vi "Get.vi"(9 "Idx (0)":i32, 10 "key":string, 11 "Keys":map{string, string[]}(c390)) -> (0 "Values out":string[](array[string]), 1 "Value out":string, 2 "Found?":bool)   [LabVIEW 2021, in "HttpServer.lvlib"]
uses:
  HttpServer.lvlib
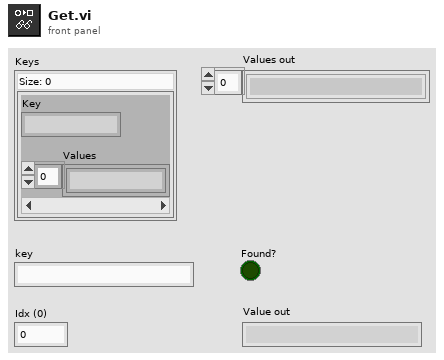
[diagram p1: front panel]
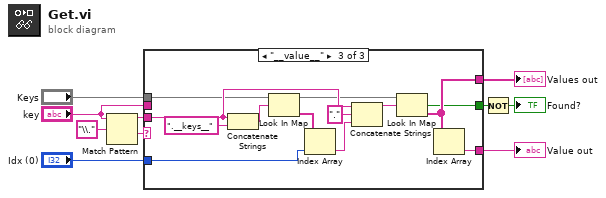
[diagram p0: block diagram]
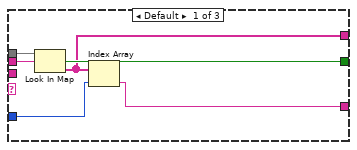
[diagram p2: hidden frame]
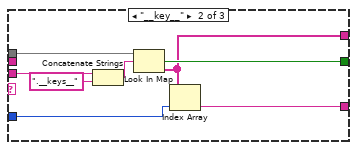
[diagram p3: hidden frame]
diagram:
  n1 = Match Pattern(string="key", regular expression="\\.") -> (before substring=w8:string, after substring=w9:string)  [unwired: 1 in, 2 out]
  n2 = case shown="\"__value__\"" w9 {
    tunnel: [w16 w24 w28] -> w4
    tunnel: "Idx (0)" -> [w14 w23 w27]
    tunnel: "Keys" -> [w15 w22 w31]
    tunnel: "key" -> [w13 _ _]
    tunnel: w8 -> [_ w19 w33]
    tunnel: [w12 w18 w25] -> w3
    tunnel: [w11 w17 w26] -> w1
    frame Default {
      n3 = Look In Map(map=w15, key=w13) -> (key not found?=w12:bool, value=w11:string[])  [unwired: 1 in]
      n4 = Index Array(array=w11, index=w14) -> (element=w16:string)
    }
    frame "__key__" {
      n5 = Concatenate Strings(w19, ".__keys__" ("string")) -> (w20:string)
      n6 = Look In Map(map=w22, key=w20) -> (key not found?=w18:bool, value=w17:string[])  [unwired: 1 in]
      n7 = Index Array(array=w17, index=w23) -> (element=w24:string)
    }
    frame "__value__" {
      n8 = Concatenate Strings(w33, ".__keys__" ("string")) -> (w35:string)
      n9 = Look In Map(map=w31, key=w35) -> (value=w34:string[])  [unwired: 1 in, 1 out]
      n10 = Index Array(array=w34, index=w27) -> (element=w29:string)
      n11 = Concatenate Strings(w33, "." ("string"), w29) -> (w30:string)
      n12 = Look In Map(map=w31, key=w30) -> (key not found?=w25:bool, value=w26:string[])  [unwired: 1 in]
      n13 = Index Array(array=w26) -> (element=w28:string)  [unwired: 1 in]
    }
  }
  "Value out" <- w4
  "Values out" <- w1
  n14 = Not(x=w3) -> (.not. x?=→"Found?":bool)
